vi "DestroyTopic.vi"(8 "error in (no error)":errorcluster, 10 "Topic Actor":string, 11 "Message Broker in":refnum<class "Message Broker.lvclass">) -> (0 "error out":errorcluster, 2 "Found?":bool, 3 "Message Broker out":refnum<class "Message Broker.lvclass">)   [LabVIEW 2016, in "Stream Mediator.lvlib" / "Message Broker.lvclass"]
doc: "--\nCopyright © 2017 Composed SystemsI All rights reserved.\n\nAuthor: Jon McBee <jon.mcbee@composed.io>\n\nThis library is provided \"AS IS\" ,WITHOUT WARRANTIES OR\nCONDITIONS OF ANY KIND, either express or implied.\n\nComposed Systems -- composed.io\n\nStream 0.0.1.1\nJon McBee - Composed Systems\nCopyright (c) 2017, Composed Systems"
uses:
  <userlib>/Composed Systems/Stream/Mediator/Classes/Message Broker/Message Broker.lvclass
  <userlib>/Composed Systems/Stream/Mediator/Classes/Message Broker/Message Broker.lvclass/Message Broker.ctl
  <userlib>/Composed Systems/Stream/Mediator/Classes/Topic Actor Stop Command/Topic Actor Stop Command.lvclass
  C:/Program Files (x86)/National Instruments/LabVIEW 2016/user.lib/Composed Systems/Stream/Mediator/Classes/Message Interface/Message Interface.lvclass
  <userlib>/Composed Systems/Stream/Mediator/Classes/Message Transport Interface/Message Priority.ctl
  <userlib>/Composed Systems/Stream/Mediator/Classes/Message Transport Queue/Message Transport Queue.lvclass
  <userlib>/Composed Systems/Stream/Mediator/Classes/Topic Actor Look Up Table/Topic Actor Look Up Table.lvclass
  <userlib>/Composed Systems/Stream/Mediator/Classes/Topic Actor Descriptor/Topic Actor Descriptor.lvclass
  <userlib>/Composed Systems/Stream/Mediator/Classes/Message Transport Interface/Message Transport Interface.lvclass
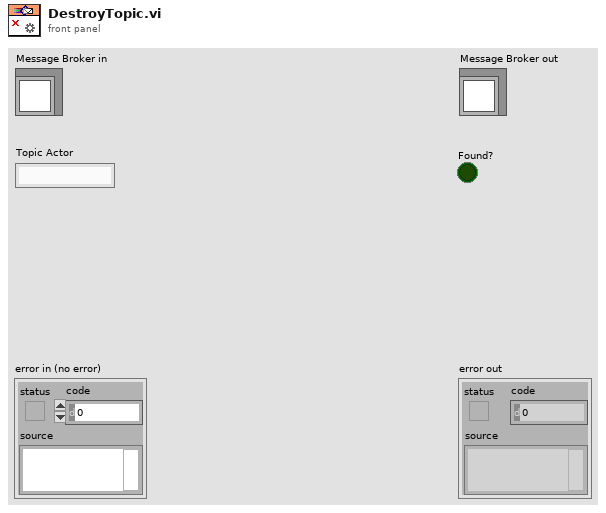
[diagram p1: front panel]
types:
  T1 = typedef "Stream Mediator.lvlib/Message Transport Interface.lvclass/Message Priority.ctl" = enum16{"Normal", "High"}
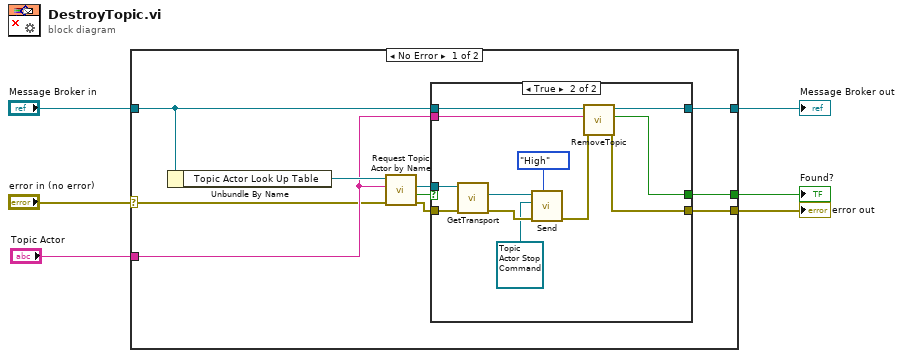
[diagram p0: block diagram]
diagram:
  n1 = case shown="No Error" "error in (no error)" {
    selector: "error in (no error)" -> [w8 w33]
    tunnel: [w7 w33] -> w5
    tunnel: [w16 w32] -> w3
    tunnel: "Message Broker in" -> [w15 w32]
    tunnel: "Topic Actor" -> [w10 _]
    tunnel: [w9 _] -> w1
    frame No Error {
      n2 = Unbundle By Name(w15) -> ("Topic Actor Look Up Table"=w14:refnum<class "Topic Actor Look Up Table.lvclass">)
      n3 = call <userlib>:"Request Topic Actor by Name.vi"("error in (no error)"=w8, "Topic Actor"=w10, "Topic Actor Look Up Table in"=w14) -> ("error out"=w11:errorcluster, "Found?"=w12:bool, "Topic Actor Descriptor"=w13:refnum<class "Topic Actor Descriptor.lvclass">)  [unwired: 5 in, 1 out]
      n4 = case shown="True" w12 {
        selector: w12 -> [w19 _]
        tunnel: [w17 w27] -> w16
        tunnel: w15 -> [w17 w26]
        tunnel: w13 -> [_ w25]
        tunnel: w11 -> [w18 w24]
        tunnel: w10 -> [_ w22]
        tunnel: [w19 w21] -> w9
        tunnel: [w18 w20] -> w7
        frame False {
        }
        frame True {
          n5 = call <userlib>:"GetTransport.vi"("error in (no error)"=w24, "Topic Actor Descriptor in"=w25) -> ("error out"=w30:errorcluster, "Transport"=w31:refnum<class "Message Transport Queue.lvclass">)  [unwired: 7 in, 1 out]
          n6 = call-dynamic "Send.vi"("Message Priority"=Message_Priority."High", "error in (no error)"=w30, "Message"=refnum<class "Topic Actor Stop Command.lvclass"> refnum ("Topic Actor Stop Command.lvclass"), "Message Transport Queue in"=w31) -> ("error out"=w23:errorcluster)  [unwired: 5 in, 2 out]
          n7 = call <userlib>:"RemoveTopic.vi"("error in (no error)"=w23, "Topic Name"=w22, "Message Broker in"=w26) -> ("error out"=w20:errorcluster, "Found?"=w21:bool, "Message Broker out"=w27:refnum<class "Message Broker.lvclass">)  [unwired: 6 in]
        }
      }
    }
    frame Error {
    }
  }
  "error out" <- w5
  "Message Broker out" <- w3
  "Found?" <- w1
